vi "Extract list from Project INI file entry.vi"(8 "error in (no error)":errorcluster, 11 "Entry from INI file":string) -> (0 "error out":errorcluster, 3 "Array":string[](array[string]))   [LabVIEW 2026, in "TALOS.lvlib"]
uses:
  TALOS.lvlib
  <vilib>/AdvancedString/Delimited String to 1D String Array (string).vi
  <vilib>/Utility/error.llb/Trim Whitespace (string).vi
  <vilib>/Utility/error.llb/Trim Whitespace One-Sided.vi
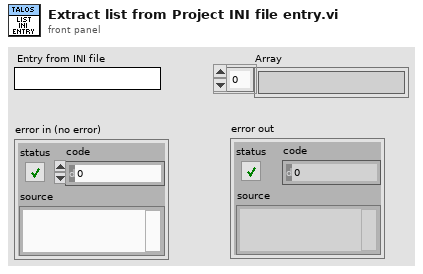
[diagram p1: front panel]
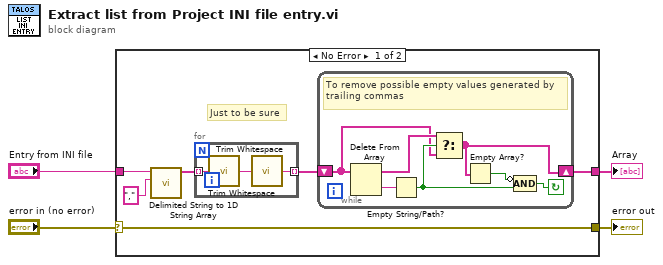
[diagram p0: block diagram]
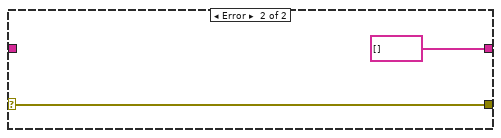
[diagram p2: hidden frame]
diagram:
  n1 = case shown="No Error" "error in (no error)" {
    selector: "error in (no error)" -> [w5 w21]
    tunnel: [w10 string[] []] -> w4
    tunnel: "Entry from INI file" -> [w9 _]
    tunnel: [w5 w21] -> w1
    frame No Error {
      # "Just to be sure"
      n2 = call-poly <vilib>:"Delimited String to 1D String Array.vi"("delimiter"=",", "delimited string"=w9) -> ("string array"=w7:string[])  [unwired: 9 in]
      n3 = for {
        tunnel: w7 -> [w20] mode=indexing
        tunnel: [w18] -> w8 mode=indexing
        n4 = call-poly <vilib>:"Trim Whitespace.vi"("string"=w20) -> ("trimmed string"=w19:string)  [unwired: 1 in]
        n5 = call-poly <vilib>:"Trim Whitespace.vi"("string"=w19) -> ("trimmed string"=w18:string)  [unwired: 1 in]
      }
      n6 = while {
        shift-right: [w12] -> w10
        shift-left: w8 -> [w14]
        stop <- w13 continue-if-true
        # "To remove possible empty values generated by trailing commas"
        n7 = Delete From Array(array=w14) -> (deleted portion=w17:string, array with subset deleted=w15:string[])  [unwired: 2 in]
        n8 = Empty String/Path?(string/path=w17) -> (empty?=w16:bool)
        n9 = Select(t=w15, s=w16, f=w14) -> (s? t:f=w12:string[])
        n10 = Empty Array?(array=w12) -> (empty?=w11:bool)
        n11 = Compound Arithmetic op=AND(invert w11, w16) -> (w13:bool)
      }
    }
    frame Error {
    }
  }
  "Array" <- w4
  "error out" <- w1
